vi "Main.vi"() -> ()   [LabVIEW 2012]
doc: "This VI is an example and a stand alone application."
uses:
  Slot.ctl
  driver/Public/Controls/64PinPGASmall.ctl
  driver/Public/Controls/64PinPGAXRay.ctl
  driver/Public/Controls/Pattern.ctl
  driver/Public/Controls/Input.ctl
  UIActionQueueElement.ctl
  UIAction.ctl
  HardwareActionQueueElement.ctl
  HardwareAction.ctl
  <vilib>/Utility/error.llb/DialogType.ctl
  driver/Virtual-PGA.lvlib
panel:
  in  "SELECT PATTEN 7":bool
  out "Card 7":T1
  in  "SELECT PATTEN 6":bool
  out "Card 6":T1
  in  "SELECT PATTEN 5":bool
  out "Card 5":T1
  in  "SELECT PATTEN 4":bool
  out "Card 4":T1
  in  "SELECT PATTEN 3":bool
  out "Card 3":T1
  in  "SELECT PATTEN 2":bool
  out "Card 2":T1
  in  "SELECT PATTEN 1":bool
  out "Card 1":T1
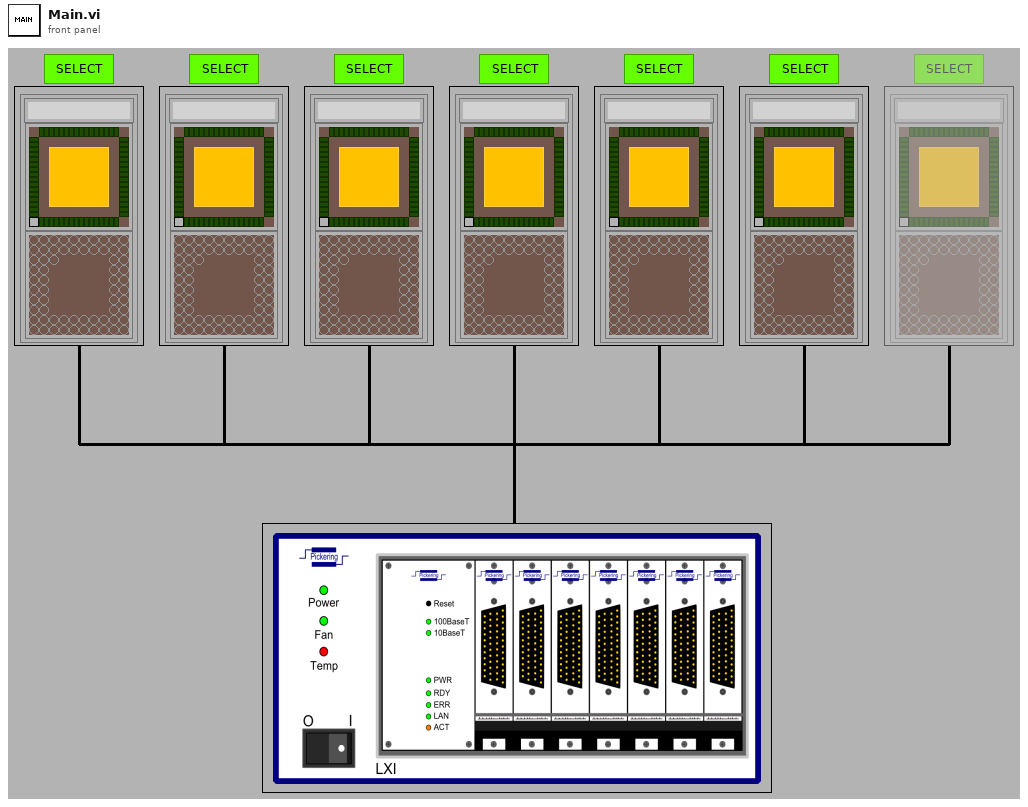
[diagram p1: front panel]
types:
  T1 = typedef "Slot.ctl" = cluster{"Patten Name":string, "PGA":T2, "XRay":T3}
  T2 = typedef "Virtual-PGA.lvlib/64PinPGASmall.ctl" = cluster{"Pad 49":bool, "Pad 50":bool, "Pad 51":bool, "Pad 52":bool, "Pad 53":bool, "Pad 54":bool, "Pad 55":bool, "Pad 56":bool, "Pad 57":bool, "Pad 58":bool, "Pad 59":bool, "Pad 60":bool, "Pad 61":bool, "Pad 62":bool, "Pad 63":bool, "Pad 64":bool, "Pad 32":bool, "Pad 31":bool, "Pad 30":bool, "Pad 29":bool, "Pad 28":bool, "Pad 27":bool, "Pad 26":bool, "Pad 25":bool, "Pad 24":bool, "Pad 23":bool, "Pad 22":bool, "Pad 21":bool, "Pad 20":bool, "Pad 19":bool, "Pad 18":bool, "Pad 17":bool, "Pad 1":bool, "Pad 2":bool, "Pad 3":bool, "Pad 4":bool, "Pad 5":bool, "Pad 6":bool, "Pad 7":bool, "Pad 8":bool, "Pad 9":bool, "Pad 10":bool, "Pad 11":bool, "Pad 12":bool, "Pad 13":bool, "Pad 14":bool, "Pad 15":bool, "Pad 16":bool, "Pad 48":bool, "Pad 47":bool, "Pad 46":bool, "Pad 45":bool, "Pad 44":bool, "Pad 43":bool, "Pad 42":bool, "Pad 41":bool, "Pad 40":bool, "Pad 39":bool, "Pad 38":bool, "Pad 37":bool, "Pad 36":bool, "Pad 35":bool, "Pad 34":bool, "Pad 33":bool}
  T3 = typedef "Virtual-PGA.lvlib/64PinPGAXRay.ctl" = cluster{"Pin 1":bool, "Pin 2":bool, "Pin 3":bool, "Pin 53":bool, "Pin 64":bool, "Pin 50":bool, "Pin 62":bool, "Pin 60":bool, "Pin 58":bool, "Pin 56":bool, "Pin 42":bool, "Pin 44":bool, "Pin 48":bool, "Pin 46":bool, "Pin 51":bool, "Pin 40":bool, "Pin 37":bool, "Pin 30":bool, "Pin 26":bool, "Pin 32":bool, "Pin 28":bool, "Pin 34":bool, "Pin 24":bool, "Pin 31":bool, "Pin 21":bool, "Pin 18":bool, "Pin 19":bool, "Pin 16":bool, "Pin 14":bool, "Pin 12":bool, "Pin 10":bool, "Pin 8":bool, "Pin 5":bool, "Pin 63":bool, "Pin 61":bool, "Pin 59":bool, "Pin 57":bool, "Pin 55":bool, "Pin 54":bool, "Pin 52":bool, "Pin 65":bool, "Pin 29":bool, "Pin 27":bool, "Pin 25":bool, "Pin 23":bool, "Pin 22":bool, "Pin 20":bool, "Pin 33":bool, "Pin 35":bool, "Pin 36":bool, "Pin 38":bool, "Pin 39":bool, "Pin 41":bool, "Pin 43":bool, "Pin 45":bool, "Pin 47":bool, "Pin 49":bool, "Pin 17":bool, "Pin 15":bool, "Pin 13":bool, "Pin 11":bool, "Pin 9":bool, "Pin 7":bool, "Pin 6":bool, "Pin 4":bool}
  T4 = typedef "Virtual-PGA.lvlib/Pattern.ctl" = cluster{"Name":string, "Description":string, "Inputs":T5[]}
  T5 = typedef "Virtual-PGA.lvlib/Input.ctl" = cluster{"ID":string, "Label":string, "Pads":u32[]}
  T6 = typedef "ActionQueues.ctl" = cluster{"UI Action":refnum<queue>, "Hardware Action":refnum<queue>}
  T7 = typedef "ExecutableConfiguration.ctl" = cluster{"Default Monitor":i32, "Center on Monitor?":bool, "IP Address":string, "Default Pattern Folder":path}
  T8 = typedef "HardwareActionQueueElement.ctl" = cluster{"State":T9, "Data":variant}
  T9 = typedef "HardwareAction.ctl" = enum16{"Initialize", "Start", "Read", "Write", "Stop", "Shutdown"}
  T10 = typedef "UIActionQueueElement.ctl" = cluster{"Action":T11, "Data":variant}
  T11 = typedef "UIAction.ctl" = enum16{"Initialize", "Connected", "Select Pattern", "Update Patterns", "Error", "Shutdown"}
  T12 = enum8{"Enabled", "Disabled", "Disabled and Grayed Out"}
  T13 = typedef "DialogType.ctl" = u16
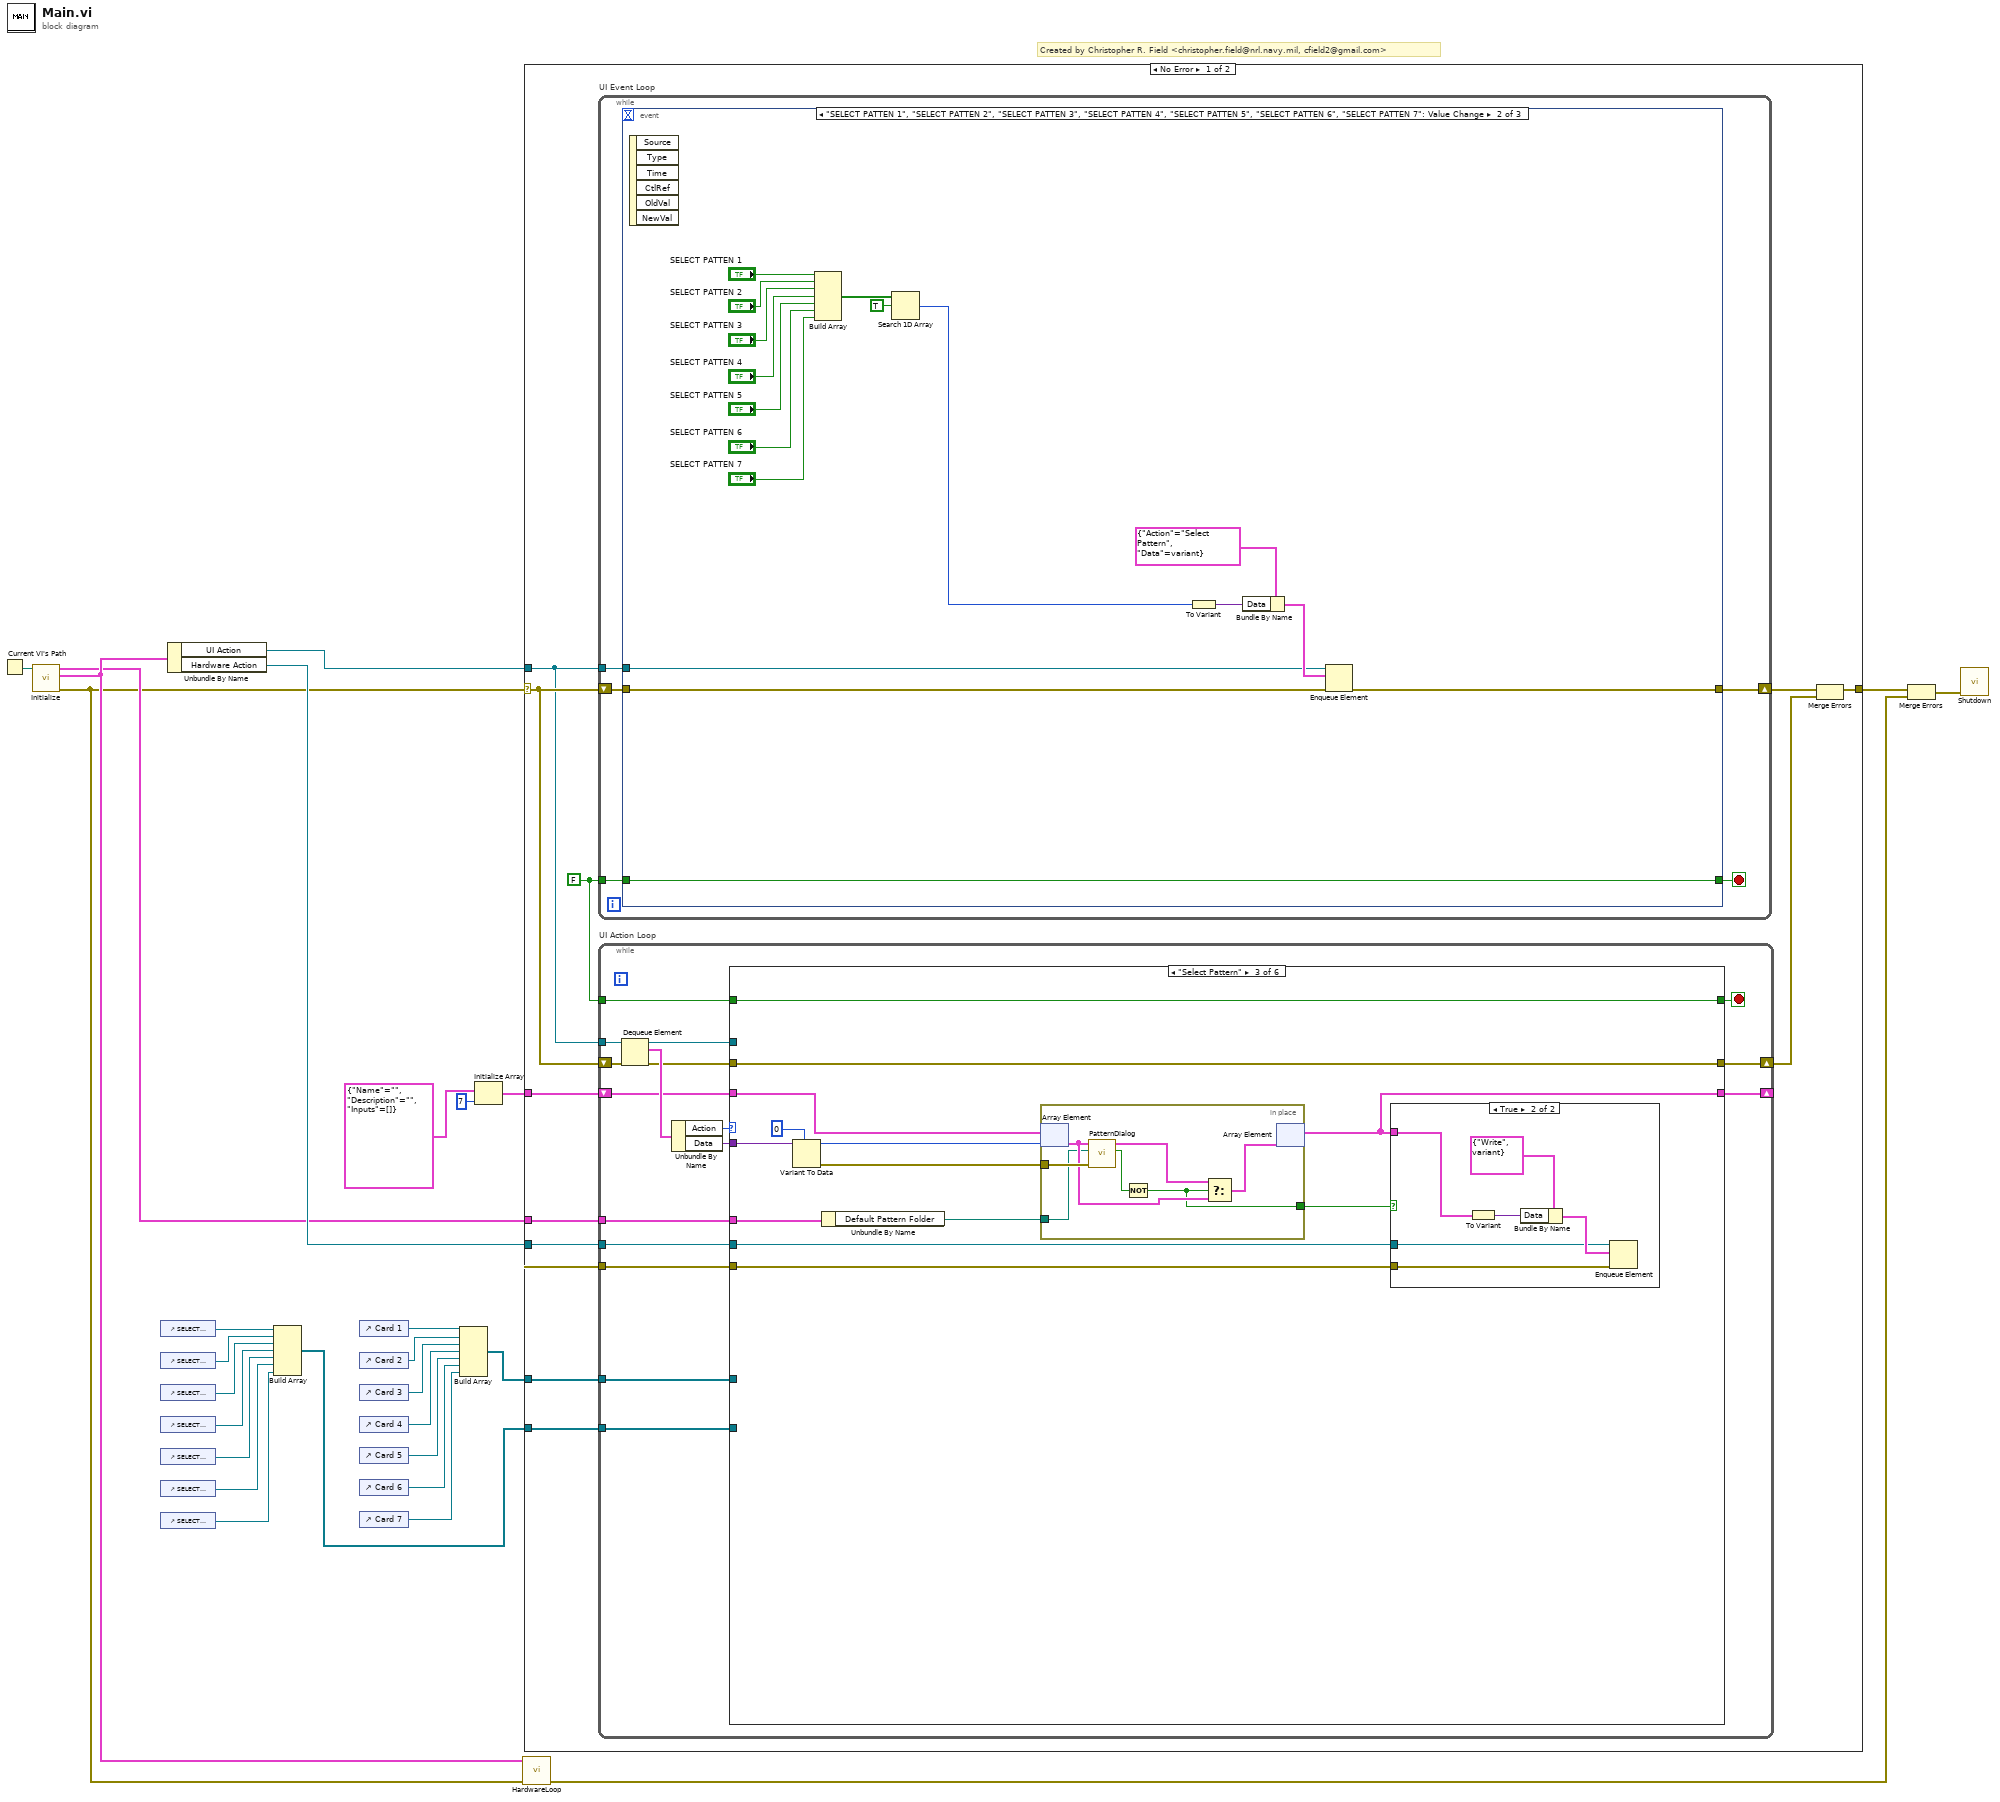
[diagram p0: block diagram]
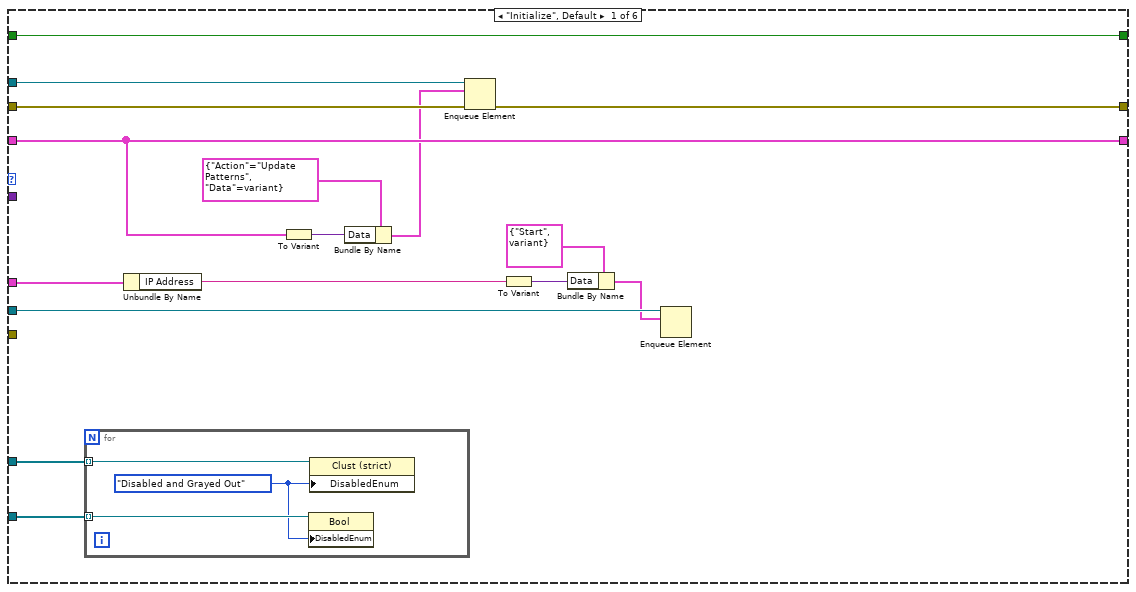
[diagram p2: hidden frame]
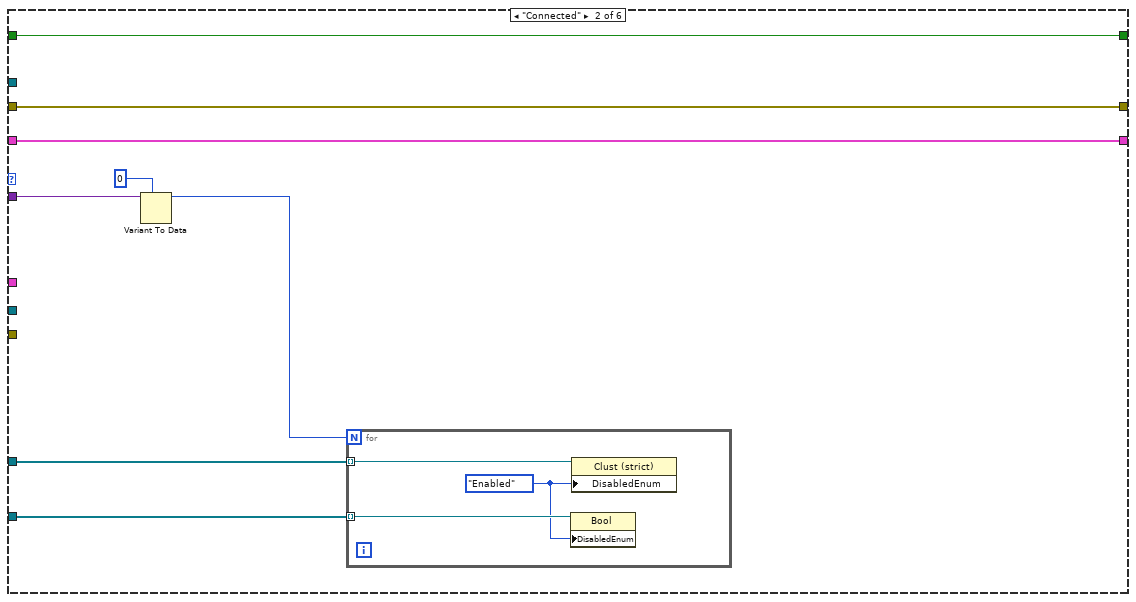
[diagram p3: hidden frame]
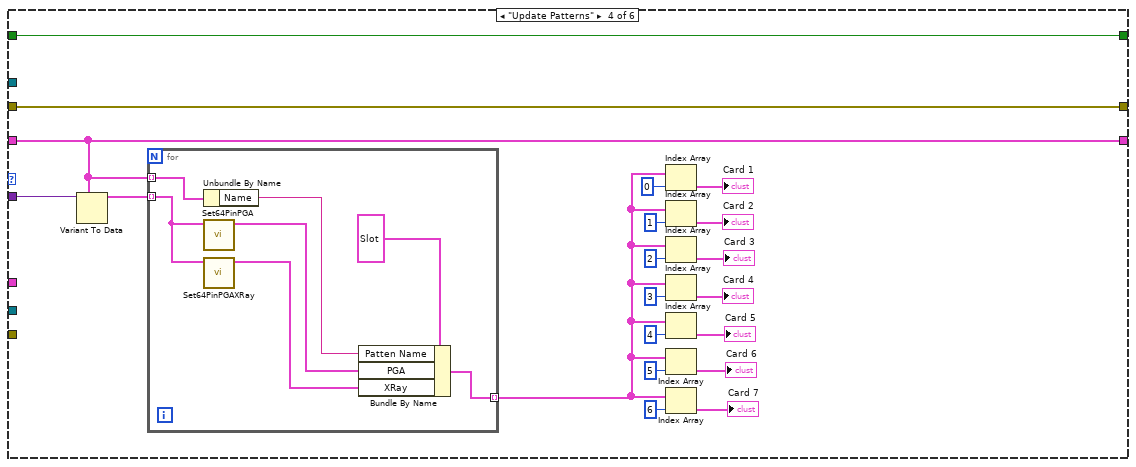
[diagram p5: hidden frame]
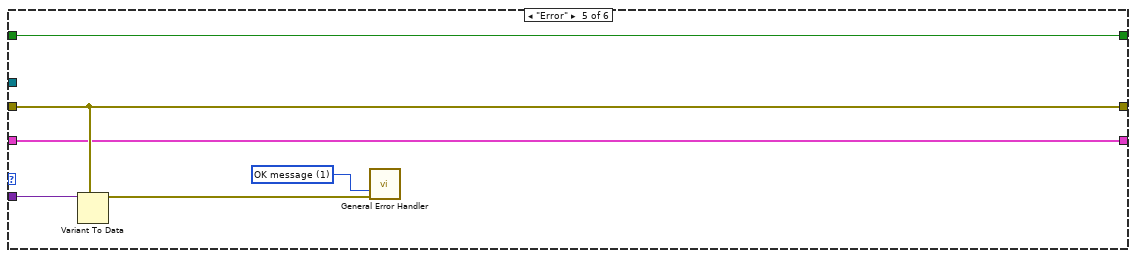
[diagram p6: hidden frame]
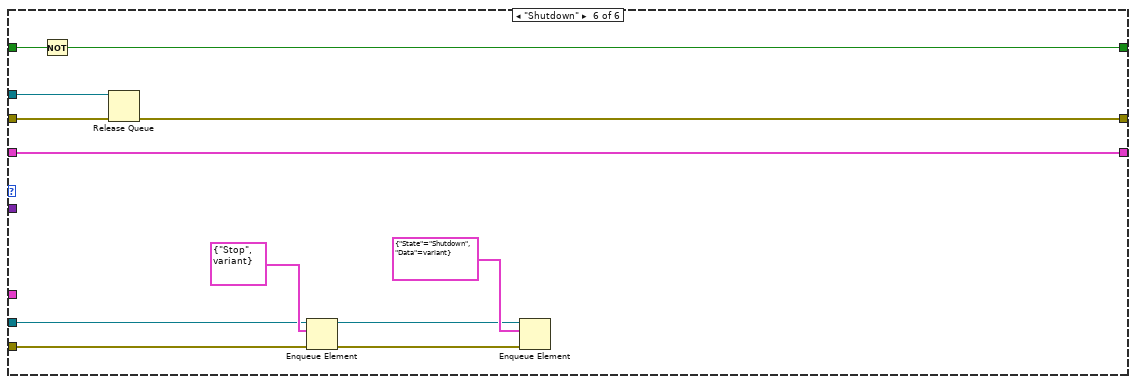
[diagram p7: hidden frame]
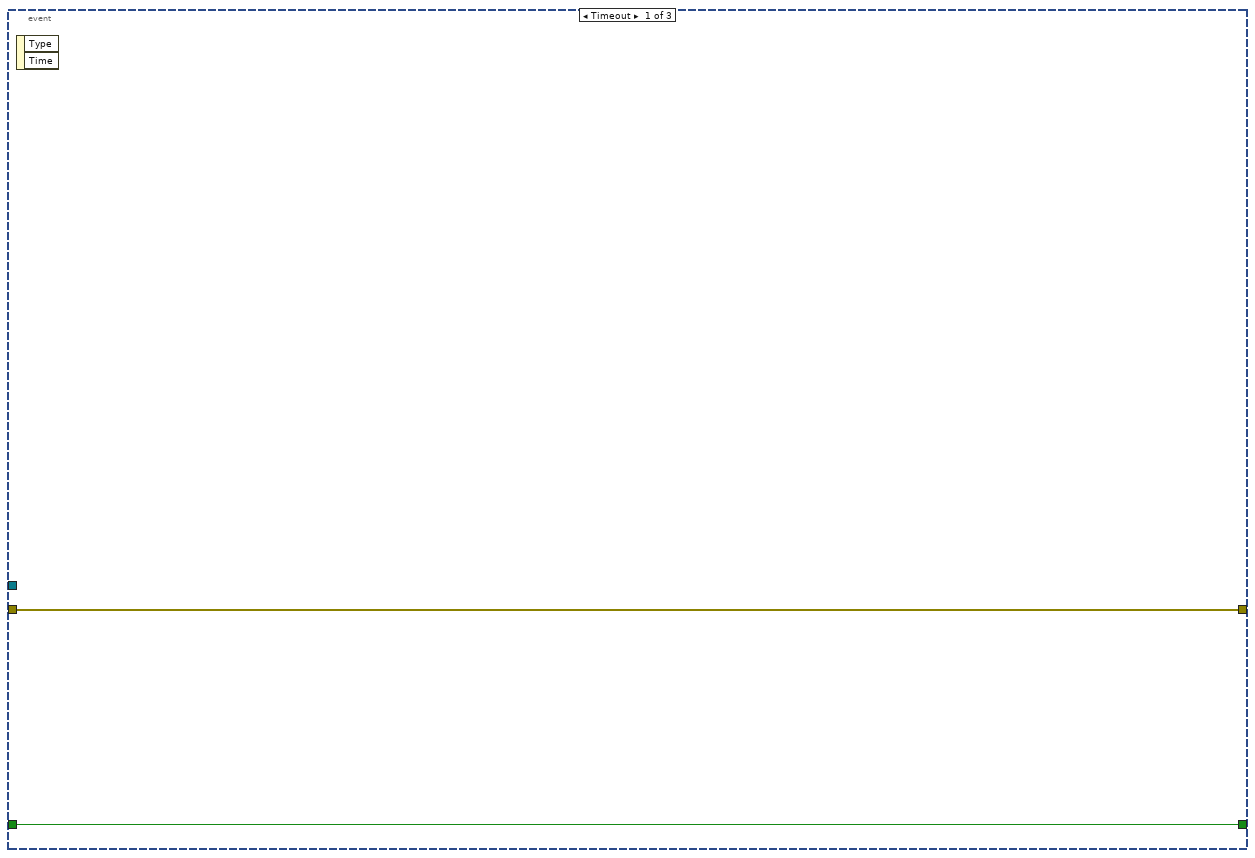
[diagram p8: hidden frame]
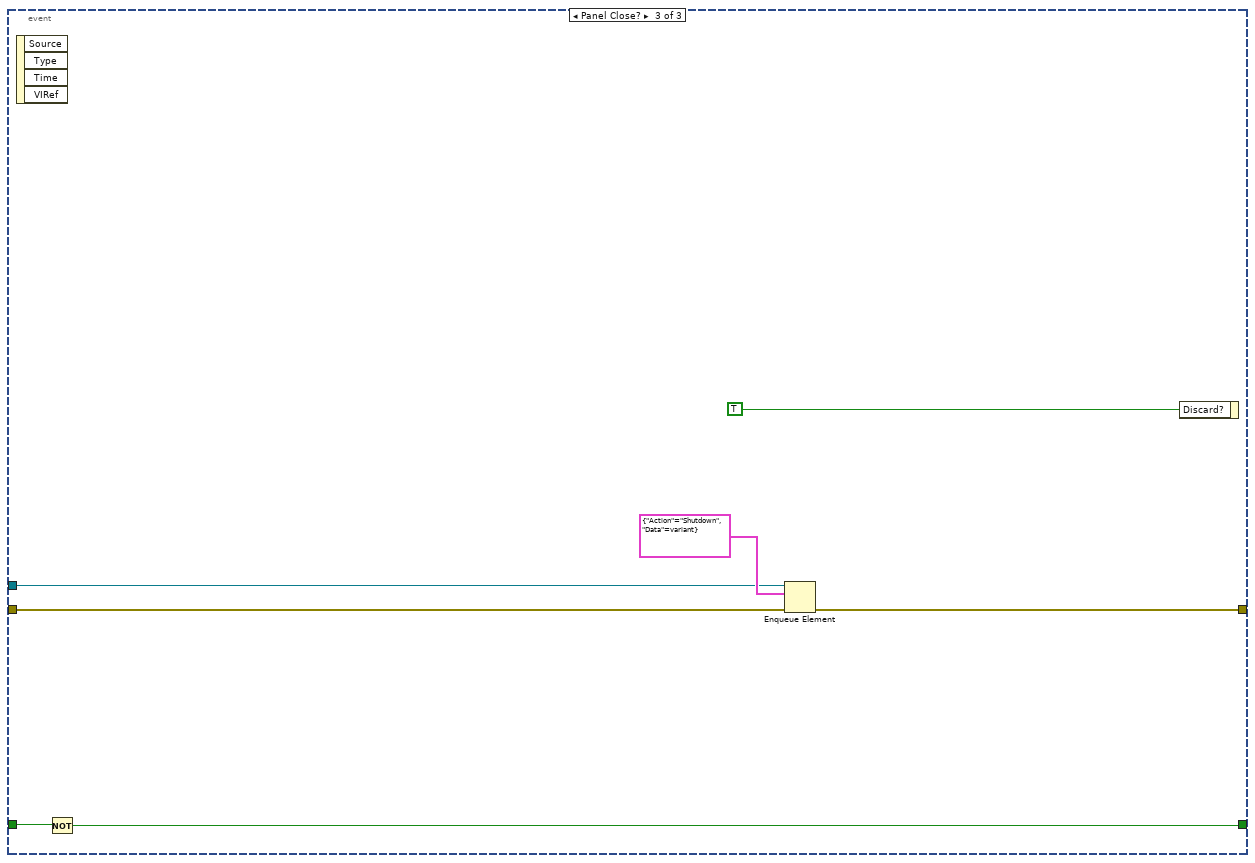
[diagram p9: hidden frame]
diagram:
  # "Created by Christopher R. Field <christopher.field@nrl.navy.mil, cfield2@gmail.com>"
  n1 = Current VI's Path() -> (path=w28:path)
  n2 = call "Initialize.vi"("VI Path"=w28) -> ("Error Out"=w1:errorcluster, "Message Queues"=w6:T6, "Executable Configuration"=w5:T7)  [unwired: 8 in]
  n3 = control-ref of="SELECT PATTEN 1"() -> (w17:refnum<vi>)
  n4 = control-ref of="SELECT PATTEN 2"() -> (w16:refnum<vi>)
  n5 = control-ref of="SELECT PATTEN 3"() -> (w15:refnum<vi>)
  n6 = control-ref of="SELECT PATTEN 4"() -> (w14:refnum<vi>)
  n7 = control-ref of="SELECT PATTEN 5"() -> (w13:refnum<vi>)
  n8 = control-ref of="SELECT PATTEN 6"() -> (w12:refnum<vi>)
  n9 = control-ref of="SELECT PATTEN 7"() -> (w11:refnum<vi>)
  n10 = Unbundle By Name(w6) -> ("UI Action"=w27:refnum<queue>, "Hardware Action"=w26:refnum<queue>)
  n11 = Build Array(w17, w16, w15, w14, w13, w12, w11) -> (w10:refnum<vi>[])
  n12 = control-ref of="Card 1"() -> (w25:refnum<vi>)
  n13 = control-ref of="Card 2"() -> (w24:refnum<vi>)
  n14 = control-ref of="Card 3"() -> (w23:refnum<vi>)
  n15 = control-ref of="Card 4"() -> (w22:refnum<vi>)
  n16 = control-ref of="Card 5"() -> (w21:refnum<vi>)
  n17 = control-ref of="Card 6"() -> (w20:refnum<vi>)
  n18 = control-ref of="Card 7"() -> (w19:refnum<vi>)
  n19 = Build Array(w25, w24, w23, w22, w21, w20, w19) -> (w18:refnum<vi>[])
  n20 = Initialize Array(T4 {"Name"="", "Description"="", "Inputs"=[]} ("Pattern"), 7 ("dimension size")) -> (w8:T4[])
  n21 = call "HardwareLoop.vi"("Error In"=w1, "Action Queues"=w6) -> ("Error Out"=w2:errorcluster)  [unwired: 9 in]
  n22 = case shown="No Error" w1 {
    selector: w1 -> [w33 w189]
    tunnel: w27 -> [w32 _]
    tunnel: w26 -> [w38 _]
    tunnel: w18 -> [w37 _]
    tunnel: w10 -> [w36 _]
    tunnel: w8 -> [w35 _]
    tunnel: w5 -> [w34 _]
    tunnel: [w29 w189] -> w4
    frame No Error {
      w39 = FALSE
      n23 = while "UI Event Loop" {
        tunnel: w39 -> [w162]
        shift-right: [w160] -> w31
        shift-left: w33 -> [w159]
        tunnel: w32 -> [w158]
        stop <- w161 stop-if-true
        n24 = event shown="[1] \"SELECT PATTEN 1\", \"SELECT PATTEN 2\", \"SELECT PATTEN 3\", \"SELECT PATTEN 4\", \"SELECT PATTEN 5\", \"SELECT PATTEN 6\", \"SELECT PATTEN 7\": Value Change" {
          selector: _ -> [_ _ _]
          dyn-events: _ -> [_ _ _]
          timeout: _ -> [_ _ _]
          tunnel: w162 -> [w164 w181 w188]
          tunnel: [w164 w181 w187] -> w161
          tunnel: w159 -> [w163 w180 w186]
          tunnel: [w163 w179 w185] -> w160
          tunnel: w158 -> [_ w165 w182]
          event Timeout {
            n25 = event-data() -> ()  [unwired: 1 in, 2 out]
          }
          event "SELECT PATTEN 1", "SELECT PATTEN 2", "SELECT PATTEN 3", "SELECT PATTEN 4", "SELECT PATTEN 5", "SELECT PATTEN 6", "SELECT PATTEN 7": Value Change {
            n26 = event-data() -> ()  [unwired: 1 in, 6 out]
            n27 = Build Array("SELECT PATTEN 1", "SELECT PATTEN 2", "SELECT PATTEN 3", "SELECT PATTEN 4", "SELECT PATTEN 5", "SELECT PATTEN 6", "SELECT PATTEN 7") -> (w168:bool[])
            n28 = Search 1D Array(1D array=w168, element=TRUE) -> (index of element=w166:i32)  [unwired: 1 in]
            n29 = To Variant(anything=w166) -> (Variant=w177:variant)
            n30 = Bundle By Name(cluster=T10 {"Action"=enum."Select Pattern", "Data"=variant} ("User Interface Queue Element"), "Data"=w177) -> (w176:T10)
            n31 = Enqueue Element(queue=w165, element=w176, error in (no error)=w180) -> (error out=w179:errorcluster)  [unwired: 1 in, 2 out]
          }
          event Panel Close? {
            n32 = event-data() -> ()  [unwired: 1 in, 4 out]
            n33 = Not(x=w188) -> (.not. x?=w187:bool)
            n34 = Enqueue Element(queue=w182, element=T10 {"Action"=enum."Shutdown", "Data"=variant}, error in (no error)=w186) -> (error out=w185:errorcluster)  [unwired: 1 in, 2 out]
            n35 = event-data("Discard?"=TRUE) -> ()  [unwired: 1 in, 1 out]
          }
        }
      }
      n36 = while "UI Action Loop" {
        tunnel: w39 -> [w50]
        shift-right: [w48] -> w30
        shift-left: w33 -> [w56]
        shift-right: [w45] -> _
        shift-left: w35 -> [w47]
        tunnel: w38 -> [w46]
        tunnel: w37 -> [w44]
        tunnel: w36 -> [w43]
        tunnel: w33 -> [w42]
        tunnel: w34 -> [w41]
        tunnel: w32 -> [w40]
        stop <- w49 stop-if-true
        n37 = Dequeue Element(queue=w40, error in (no error)=w56) -> (queue out=w53:refnum<queue>, element=w55:T10, error out=w54:errorcluster)  [unwired: 1 in, 1 out]
        n38 = Unbundle By Name(w55) -> ("Action"=w52:T11, "Data"=w51:variant)
        n39 = case shown="\"Select Pattern\"" w52 {
          tunnel: w54 -> [w68 w82 w98 w132 w143 w147]
          tunnel: w53 -> [w69 _ _ _ _ w148]
          tunnel: w51 -> [_ w78 w97 w130 w144 _]
          tunnel: w50 -> [w72 w83 w99 w131 w145 w157]
          tunnel: [w72 w83 w99 w131 w145 w156] -> w49
          tunnel: [w67 w82 w98 w132 w143 w146] -> w48
          tunnel: w47 -> [w64 w81 w95 w113 w142 w155]
          tunnel: w46 -> [w62 _ w92 _ _ w149]
          tunnel: [w64 w81 w93 w113 w142 w155] -> w45
          tunnel: w44 -> [w71 w80 _ _ _ _]
          tunnel: w43 -> [w70 w79 _ _ _ _]
          tunnel: w42 -> [_ _ w91 _ _ w153]
          tunnel: w41 -> [w59 _ w88 _ _ _]
          frame "Initialize", Default {
            n40 = for {
              tunnel: w71 -> [w75] mode=indexing
              tunnel: w70 -> [w74] mode=indexing
              w73 = T12."Disabled and Grayed Out" ("Disabled")
              n41 = property class="Bool"(reference=w74, "DisabledEnum"=w73) -> ()  [unwired: 1 in, 2 out]
              n42 = property class="Clust (strict)"(reference=w75, "DisabledEnum"=w73) -> ()  [unwired: 1 in, 2 out]
            }
            n43 = Unbundle By Name(w59) -> ("IP Address"=w58:string)
            n44 = To Variant(anything=w64) -> (Variant=w65:variant)
            n45 = Bundle By Name(cluster=T10 {"Action"=enum."Update Patterns", "Data"=variant} ("element"), "Data"=w65) -> (w63:T10)
            n46 = Enqueue Element(queue=w69, element=w63, error in (no error)=w68) -> (error out=w67:errorcluster)  [unwired: 1 in, 2 out]
            n47 = To Variant(anything=w58) -> (Variant=w60:variant)
            n48 = Bundle By Name(cluster=T8 {"State"=enum."Start", "Data"=variant} ("element"), "Data"=w60) -> (w57:T8)
            n49 = Enqueue Element(queue=w62, element=w57) -> ()  [unwired: 2 in, 3 out]
          }
          frame "Connected" {
            n50 = Variant To Data(type=0 ("size(s)"), Variant=w78) -> (data=w76:i32)  [unwired: 1 in, 1 out]
            n51 = for {
              N: w76 -> [_]
              tunnel: w80 -> [w86] mode=indexing
              tunnel: w79 -> [w85] mode=indexing
              w84 = T12."Enabled" ("Disabled")
              n52 = property class="Bool"(reference=w85, "DisabledEnum"=w84) -> ()  [unwired: 1 in, 2 out]
              n53 = property class="Clust (strict)"(reference=w86, "DisabledEnum"=w84) -> ()  [unwired: 1 in, 2 out]
            }
          }
          frame "Select Pattern" {
            n54 = Variant To Data(type=0 ("index of element"), Variant=w97) -> (data=w94:i32, error out=w90:errorcluster)  [unwired: 1 in]
            n55 = Unbundle By Name(w88) -> ("Default Pattern Folder"=w87:path)
            n56 = in-place {
              in-place-border: w90 -> [w111]
              in-place-border: [w107] -> w89
              in-place-border: w87 -> [w106]
              n57 = in-place-array #1(w95, w94) -> (w109:T4)
              n58 = call "PatternDialog.vi"("Error In"=w111, "Default Pattern Folder"=w106, "Pattern In"=w109) -> ("Cancelled?"=w112:bool, "Pattern Out"=w110:T4)  [unwired: 6 in, 1 out]
              n59 = Not(x=w112) -> (.not. x?=w107:bool)
              n60 = Select(t=w110, s=w107, f=w109) -> (s? t:f=w108:T4)
              n61 = in-place-array #1(w108) -> (w93:T4[])  [unwired: 1 out]
            }
            n62 = case shown="True" w89 {
              tunnel: w93 -> [_ w102]
              tunnel: w92 -> [_ w100]
              tunnel: w91 -> [_ w101]
              frame False {
              }
              frame True {
                n63 = To Variant(anything=w102) -> (Variant=w103:variant)
                n64 = Bundle By Name(cluster=T8 {"State"=enum."Write", "Data"=variant} ("Acquisition Queue Element"), "Data"=w103) -> (w104:T8)
                n65 = Enqueue Element(queue=w100, element=w104, error in (no error)=w101) -> ()  [unwired: 1 in, 3 out]
              }
            }
          }
          frame "Update Patterns" {
            n66 = Variant To Data(type=w113, Variant=w130) -> (data=w129:T4[])  [unwired: 1 in, 1 out]
            n67 = for {
              tunnel: w129 -> [w134] mode=indexing
              tunnel: [w135] -> w114 mode=indexing
              tunnel: w113 -> [w133] mode=indexing
              n68 = Unbundle By Name(w133) -> ("Name"=w139:string)
              n69 = call "Set64PinPGA.vi"("Pattern"=w134) -> ("64-Pin PGA"=w138:T2)  [unwired: 10 in]
              n70 = call "Set64PinPGAXRay.vi"("Pattern"=w134) -> ("X-Ray PGA"=w137:T3)  [unwired: 10 in]
              n71 = Bundle By Name(cluster=T1 {"Patten Name"="", "PGA"={"Pad 49"=FALSE, "Pad 50"=FALSE, "Pad 51"=FALSE, "Pad 52"=FALSE, "Pad 53"=FALSE, "Pad 54"=FALSE, "Pad 55"=FALSE, "Pad 56"=FALSE, "Pad 57"=FALSE, "Pad 58"=FALSE, "Pad 59"=FALSE, "Pad 60"=FALSE, "Pad 61"=FALSE, "Pad 62"=FALSE, "Pad 63"=FALSE, "Pad 64"=FALSE, "Pad 32"=FALSE, "Pad 31"=FALSE, "Pad 30"=FALSE, "Pad 29"=FALSE, "Pad 28"=FALSE, "Pad 27"=FALSE, "Pad 26"=FALSE, "Pad 25"=FALSE, "Pad 24"=FALSE, "Pad 23"=FALSE, "Pad 22"=FALSE, "Pad 21"=FALSE, "Pad 20"=FALSE, "Pad 19"=FALSE, "Pad 18"=FALSE, "Pad 17"=FALSE, "Pad 1"=FALSE, "Pad 2"=FALSE, "Pad 3"=FALSE, "Pad 4"=FALSE, "Pad 5"=FALSE, "Pad 6"=FALSE, "Pad 7"=FALSE, "Pad 8"=FALSE, "Pad 9"=FALSE, "Pad 10"=FALSE, "Pad 11"=FALSE, "Pad 12"=FALSE, "Pad 13"=FALSE, "Pad 14"=FALSE, "Pad 15"=FALSE, "Pad 16"=FALSE, "Pad 48"=FALSE, "Pad 47"=FALSE, "Pad 46"=FALSE, "Pad 45"=FALSE, "Pad 44"=FALSE, "Pad 43"=FALSE, "Pad 42"=FALSE, "Pad 41"=FALSE, "Pad 40"=FALSE, "Pad 39"=FALSE, "Pad 38"=FALSE, "Pad 37"=FALSE, "Pad 36"=FALSE, "Pad 35"=FALSE, "Pad 34"=FALSE, "Pad 33"=FALSE}, "XRay"={"Pin 1"=FALSE, "Pin 2"=FALSE, "Pin 3"=FALSE, "Pin 53"=FALSE, "Pin 64"=FALSE, "Pin 50"=FALSE, "Pin 62"=FALSE, "Pin 60"=FALSE, "Pin 58"=FALSE, "Pin 56"=FALSE, "Pin 42"=FALSE, "Pin 44"=FALSE, "Pin 48"=FALSE, "Pin 46"=FALSE, "Pin 51"=FALSE, "Pin 40"=FALSE, "Pin 37"=FALSE, "Pin 30"=FALSE, "Pin 26"=FALSE, "Pin 32"=FALSE, "Pin 28"=FALSE, "Pin 34"=FALSE, "Pin 24"=FALSE, "Pin 31"=FALSE, "Pin 21"=FALSE, "Pin 18"=FALSE, "Pin 19"=FALSE, "Pin 16"=FALSE, "Pin 14"=FALSE, "Pin 12"=FALSE, "Pin 10"=FALSE, "Pin 8"=FALSE, "Pin 5"=FALSE, "Pin 63"=FALSE, "Pin 61"=FALSE, "Pin 59"=FALSE, "Pin 57"=FALSE, "Pin 55"=FALSE, "Pin 54"=FALSE, "Pin 52"=FALSE, "Pin 65"=FALSE, "Pin 29"=FALSE, "Pin 27"=FALSE, "Pin 25"=FALSE, "Pin 23"=FALSE, "Pin 22"=FALSE, "Pin 20"=FALSE, "Pin 33"=FALSE, "Pin 35"=FALSE, "Pin 36"=FALSE, "Pin 38"=FALSE, "Pin 39"=FALSE, "Pin 41"=FALSE, "Pin 43"=FALSE, "Pin 45"=FALSE, "Pin 47"=FALSE, "Pin 49"=FALSE, "Pin 17"=FALSE, "Pin 15"=FALSE, "Pin 13"=FALSE, "Pin 11"=FALSE, "Pin 9"=FALSE, "Pin 7"=FALSE, "Pin 6"=FALSE, "Pin 4"=FALSE}} ("Slot"), "Patten Name"=w139, "PGA"=w138, "XRay"=w137) -> (w135:T1)
            }
            n72 = Index Array(array=w114, index=0) -> (element=→"Card 1":T1)
            n73 = Index Array(array=w114, index=1) -> (element=→"Card 2":T1)
            n74 = Index Array(array=w114, index=2) -> (element=→"Card 3":T1)
            n75 = Index Array(array=w114, index=3) -> (element=→"Card 4":T1)
            n76 = Index Array(array=w114, index=4) -> (element=→"Card 5":T1)
            n77 = Index Array(array=w114, index=5) -> (element=→"Card 6":T1)
            n78 = Index Array(array=w114, index=6) -> (element=→"Card 7":T1)
          }
          frame "Error" {
            w141 = T13 1 items=["no dialog", "OK message", "continue or stop message", "OK message + warnings", "continue/stop + warnings"] ("type of dialog (OK msg:1)")
            n79 = Variant To Data(type=w143, Variant=w144) -> (data=w140:errorcluster)  [unwired: 1 in, 1 out]
            n80 = call <vilib>:"General Error Handler.vi"("type of dialog (OK msg:1)"=w141, "error in (no error)"=w140) -> ()  [unwired: 9 in, 5 out]
          }
          frame "Shutdown" {
            n81 = Not(x=w157) -> (.not. x?=w156:bool)
            n82 = Release Queue(queue=w148, error in (no error)=w147) -> (error out=w146:errorcluster)  [unwired: 1 in, 2 out]
            n83 = Enqueue Element(queue=w149, element=T8 {"State"=enum."Stop", "Data"=variant}, error in (no error)=w153) -> (queue out=w151:refnum<queue>, error out=w152:errorcluster)  [unwired: 1 in, 1 out]
            n84 = Enqueue Element(queue=w151, element=T8 {"State"=enum."Shutdown", "Data"=variant} ("Acquisition Queue Element"), error in (no error)=w152) -> ()  [unwired: 1 in, 3 out]
          }
        }
      }
      n85 = Merge Errors(w31, w30) -> (w29:errorcluster)
    }
    frame Error {
    }
  }
  n86 = Merge Errors(w4, w2) -> (w3:errorcluster)
  n87 = call "Shutdown.vi"("Error In"=w3) -> ()  [unwired: 11 in]
